vi "Contex Menu Selection.vi"(8 "error in (no error)":errorcluster, 10 "MenuItem":string, 11 "HIJ Vision Display in":refnum<class "HIJ Vision Display.lvclass">) -> (0 "error out":errorcluster, 3 "HIJ Vision Display out":refnum<class "HIJ Vision Display.lvclass">)   [LabVIEW 2014, in "HIJ Vision Display.lvlib" / "HIJ Vision Display.lvclass"]
uses:
  HIJ Vision Display.lvclass
  HIJ Vision Display.lvclass/HIJ Vision Display.ctl
  Read Display ref.vi
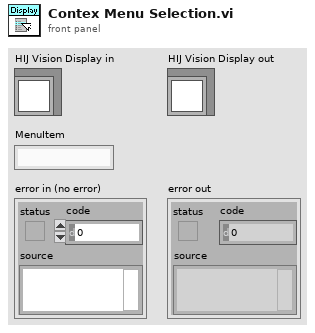
[diagram p1: front panel]
types:
  T1 = cluster{"Global Rectangle":i32[], "Contours":cluster{"Contour Type":u32, "ROI Type":u32, "Points":i32[]}[]}
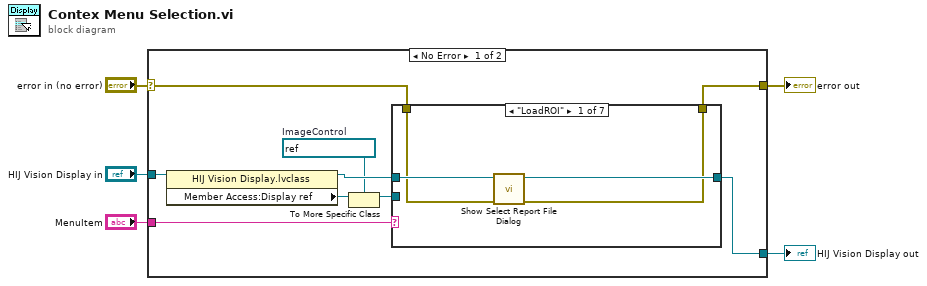
[diagram p0: block diagram]
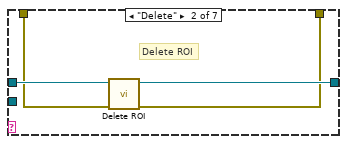
[diagram p2: hidden frame]
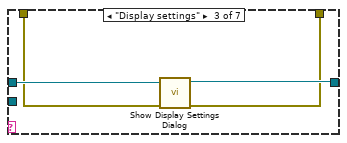
[diagram p3: hidden frame]
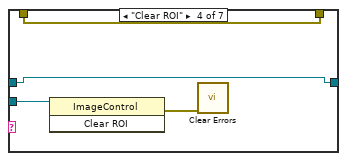
[diagram p4: hidden frame]
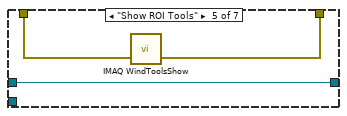
[diagram p5: hidden frame]
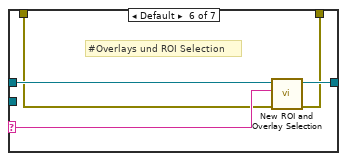
[diagram p6: hidden frame]
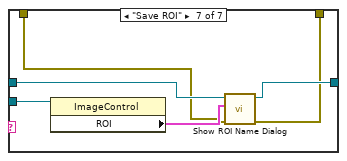
[diagram p7: hidden frame]
diagram:
  n1 = case shown="No Error" "error in (no error)" {
    selector: "error in (no error)" -> [w8 w46]
    tunnel: [w7 w46] -> w4
    tunnel: [w9 w45] -> w2
    tunnel: "HIJ Vision Display in" -> [w13 w45]
    tunnel: "MenuItem" -> [w14 _]
    frame No Error {
      w6 = refnum<vi> refnum  # ImageControl
      n2 = property class="HIJ Vision Display.lvclass"(reference=w13) -> (reference out=w10:refnum<class "HIJ Vision Display.lvclass">, "Member Access:Display ref"=w12:refnum<vi>)  [unwired: 1 in, 1 out]
      n3 = To More Specific Class(target class=w6, reference=w12) -> (specific class reference=w11:refnum<vi>)  [unwired: 1 in, 1 out]
      n4 = case shown="\"LoadROI\"" w14 {
        selector: w14 -> [_ _ _ _ _ w36 _]
        tunnel: w11 -> [_ _ _ w29 _ _ w44]
        tunnel: w10 -> [w18 w22 w26 w28 w33 w38 w43]
        tunnel: [w17 w20 w25 w28 w33 w37 w42] -> w9
        tunnel: w8 -> [w16 w21 w24 w27 w32 w35 w40]
        tunnel: [w15 w19 w23 w27 w31 w34 w39] -> w7
        frame "LoadROI" {
          n5 = call "Show Select Report File Dialog.vi"("error in (no error)"=w16, "IMAQ Display in"=w18) -> ("error out"=w15:errorcluster, "IMAQ Display out"=w17:refnum<class "HIJ Vision Display.lvclass">)  [unwired: 8 in]
        }
        frame "Delete" {
          # "Delete ROI"
          n6 = call "Delete ROI.vi"("error in (no error)"=w21, "IMAQ Display in"=w22) -> ("error out"=w19:errorcluster, "IMAQ Display out"=w20:refnum<class "HIJ Vision Display.lvclass">)  [unwired: 8 in]
        }
        frame "Display settings" {
          n7 = call "Show Display Settings Dialog.vi"("error in (no error)"=w24, "IMAQ Display in"=w26) -> ("error out"=w23:errorcluster, "IMAQ Display out"=w25:refnum<class "HIJ Vision Display.lvclass">)  [unwired: 8 in]
        }
        frame "Clear ROI" {
          n8 = invoke on="Invoke Node" class="ImageControl" method="Clear ROI"(reference=w29) -> (error out=w30:errorcluster)  [unwired: 2 in, 2 out]
          n9 = call <vilib>:"Clear Errors.vi"("error in (no error)"=w30) -> ()  [unwired: 5 in, 2 out]
        }
        frame "Show ROI Tools" {
          n10 = call "IMAQ WindToolsShow"("error in (no error)"=w32) -> ("error out"=w31:errorcluster)  [unwired: 4 in, 1 out]
        }
        frame Default {
          # "#Overlays und ROI Selection"
          n11 = call-dynamic "New ROI and Overlay Selection.vi"("error in (no error)"=w35, "ItemTag"=w36, "IMAQ Display in"=w38) -> ("error out"=w34:errorcluster, "IMAQ Display out"=w37:refnum<class "HIJ Vision Display.lvclass">)  [unwired: 7 in]
        }
        frame "Save ROI" {
          n12 = property on="Property Node" class="ImageControl"(reference=w44) -> ("ROI"=w41:T1)  [unwired: 1 in, 2 out]
          n13 = call-dynamic "Show ROI Name Dialog.vi"("error in (no error)"=w40, "ROI Descriptor"=w41, "IMAQ Display in"=w43) -> ("error out"=w39:errorcluster, "IMAQ Display out"=w42:refnum<class "HIJ Vision Display.lvclass">)  [unwired: 7 in]
        }
      }
    }
    frame Error {
    }
  }
  "error out" <- w4
  "HIJ Vision Display out" <- w2
